vi "Insight_Write_Laser_Parameters_to_File.vi"(6 "Hold Data Vector":i32[](array[numeric]), 7 "Filename Preface (empty)":string, 8 "error in (no error)":errorcluster, 9 "Actual Laser Settings":T3={"Clock Rate (MHz)"=400.0, "Sample Pts"=0, "Total Sweep Pts"=0, "Total Pts Increment"=0, "Reversal Index"=0, "Sweep Efficiency (%)"=nan, "Duty Cycle (%)"=nan, "Repetition Rate (kHz)"=nan, "Sweep Rate (kHz)"=nan, "Min Wavelength (nm)"=nan, "Max Wavelength (nm)"=nan, "Power (mW)"=nan, "Power Profile"=enum."FLAT", "Edge Roll-off (dB)"=0.0, "Sample Clock Delay (nsec)"=0.0, "Sweep Start Delay (nsec)"=0.0, "Data Valid Delay (nsec)"=0.0, "Optical Freq. Step (GHz)"=0.1, "Sweep Start Trigger Edge"=enum."BOTH", "WL Sweep Direction?"=enum."Increase"}, 10 "Valid Vector":i32[](array[numeric]), 11 "Save Data Path":path=path "C:/Users/Demonstration/Documents/LabView_Applications/Projects/Insight_SPD_Acquire/laser_data") -> (0 "error out":errorcluster, 1 "Hold Data Vector Path":path=path "C:/Users/Demonstration/Documents/LabView_Applications/Projects/Insight_SPD_Acquire/laser_data", 2 "Laser Parameter Data Path":path=path "C:/Users/Demonstration/Documents/LabView_Applications/Projects/Insight_SPD_Acquire/laser_data", 3 "DVV Path":path=path "C:/Users/Demonstration/Documents/LabView_Applications/Projects/Insight_SPD_Acquire/laser_data")   [LabVIEW 2011]
doc: "Insight Photonic Solutions\n\nThis VI writes Actual Laser Settings cluster, Data Valid Vector and Hold Data Vector (aka Invalid Data Points) to Laser Parameter, DVV and Hold Data text files.\n\nUse the Filename Preface to add a specific filename descriptor like a date, time or random sequence.\n\nver 1.0 - original release\nver 1.1 - added inputs for the Hold Data Vector of hold points, writes this data to a file, and output the pathname to this file.\nver 3.5 - updated Actual Laser Settings to add Total Pts Incrementt, Reversal Index, and Sweep Rate. Also modified the formatting of the string written to the file to use the appropriate precision."
uses:
  Power_Profiles.ctl
  Start_Sweep_Trigger.ctl
  <vilib>/Utility/file.llb/Write To Spreadsheet File (I64).vi
  <vilib>/Utility/file.llb/Write To Spreadsheet File (string).vi
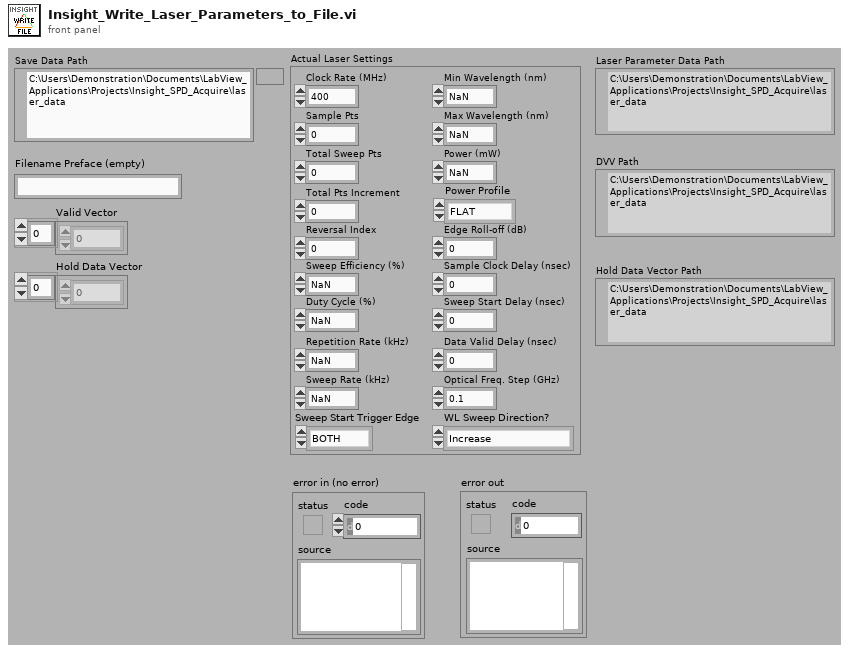
[diagram p1: front panel]
types:
  T1 = typedef "Power_Profiles.ctl" = enum16{"FLAT", "GAUSsian", "CUSTom"}
  T2 = typedef "Start_Sweep_Trigger.ctl" = enum16{"RISing", "FALLing", "BOTH"}
  T3 = cluster{"Clock Rate (MHz)":dbl, "Sample Pts":u32, "Total Sweep Pts":i32, "Total Pts Increment":i32, "Reversal Index":i32, "Sweep Efficiency (%)":dbl, "Duty Cycle (%)":dbl, "Repetition Rate (kHz)":dbl, "Sweep Rate (kHz)":dbl, "Min Wavelength (nm)":dbl, "Max Wavelength (nm)":dbl, "Power (mW)":dbl, "Power Profile":T1, "Edge Roll-off (dB)":dbl, "Sample Clock Delay (nsec)":dbl, "Sweep Start Delay (nsec)":dbl, "Data Valid Delay (nsec)":dbl, "Optical Freq. Step (GHz)":dbl, "Sweep Start Trigger Edge":T2, "WL Sweep Direction?":enum16{"Increase", "Decrease", "Bidirectional_Increase", "Bidirectional_Decrease"}}
  T4 = enum16{"Increase", "Decrease", "Bidirectional_Increase", "Bidirectional_Decrease"}
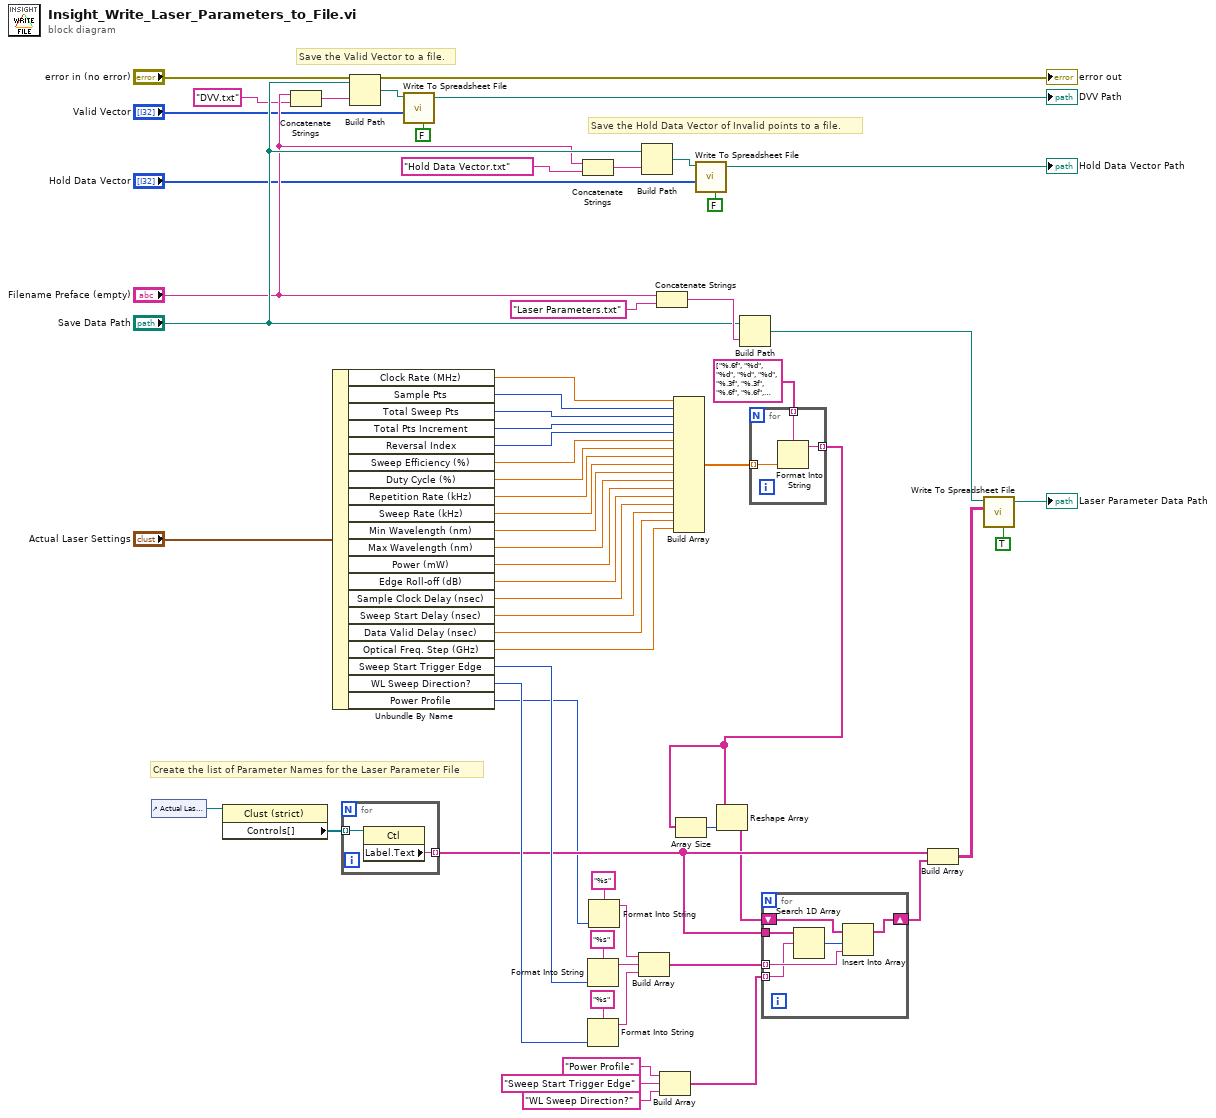
[diagram p0: block diagram]
diagram:
  # "Save the Hold Data Vector of Invalid points to a file."
  # "Save the Valid Vector to a file."
  # "Create the list of Parameter Names for the Laser Parameter File"
  n1 = control-ref of="Actual Laser Settings"() -> (w44:refnum<vi>)
  n2 = property class="Clust (strict)"(reference=w44) -> ("Controls[]"=w45:refnum<vi>[])  [unwired: 1 in, 2 out]
  n3 = Concatenate Strings("Filename Preface (empty)", "DVV.txt" ("time format string (%c)")) -> (w12:string)
  n4 = Unbundle By Name("Actual Laser Settings") -> ("Clock Rate (MHz)"=w62:dbl, "Sample Pts"=w61:u32, "Total Sweep Pts"=w60:i32, "Total Pts Increment"=w39:i32, "Reversal Index"=w38:i32, "Sweep Efficiency (%)"=w59:dbl, "Duty Cycle (%)"=w46:dbl, "Repetition Rate (kHz)"=w58:dbl, "Sweep Rate (kHz)"=w37:dbl, "Min Wavelength (nm)"=w57:dbl, "Max Wavelength (nm)"=w56:dbl, "Power (mW)"=w55:dbl, "Edge Roll-off (dB)"=w35:dbl, "Sample Clock Delay (nsec)"=w54:dbl, "Sweep Start Delay (nsec)"=w53:dbl, "Data Valid Delay (nsec)"=w52:dbl, "Optical Freq. Step (GHz)"=w51:dbl, "Sweep Start Trigger Edge"=w33:T2, "WL Sweep Direction?"=w31:T4, "Power Profile"=w2:T1)
  n5 = for {
    tunnel: w45 -> [w64] mode=indexing
    tunnel: [w63] -> w21 mode=indexing
    n6 = property class="Ctl"(reference=w64) -> ("Label.Text"=w63:string)  [unwired: 1 in, 2 out]
  }
  n7 = Build Path(base path="Save Data Path", name or relative path=w12) -> (appended path=w16:path)
  n8 = call-poly <vilib>:"Write To Spreadsheet File.vi"("transpose? (no:F)"=FALSE, "1D data"="Valid Vector", "file path (dialog if empty)"=w16) -> ("new file path (Not A Path if cancelled)"=→"DVV Path":path)  [unwired: 5 in]
  n9 = Concatenate Strings("Filename Preface (empty)", "Hold Data Vector.txt" ("time format string (%c)")) -> (w9:string)
  n10 = Format Into String(format string="%s", w33) -> (resulting string=w27:string)  [unwired: 2 in, 1 out]
  n11 = Format Into String(format string="%s", w31) -> (resulting string=w26:string)  [unwired: 2 in, 1 out]
  n12 = Format Into String(format string="%s", w2) -> (resulting string=w22:string)  [unwired: 2 in, 1 out]
  n13 = Build Array(w22, w27, w26) -> (w25:string[])
  n14 = Build Path(base path="Save Data Path", name or relative path=w9) -> (appended path=w7:path)
  n15 = Concatenate Strings("Filename Preface (empty)", "Laser Parameters.txt" ("time format string (%c)")) -> (w42:string)
  n16 = Build Array("Power Profile", "Sweep Start Trigger Edge", "WL Sweep Direction?") -> (w24:string[])
  n17 = Build Array(w62, w61, w60, w39, w38, w59, w46, w58, w37, w57, w56, w55, w35, w54, w53, w52, w51) -> (w49:dbl[])
  n18 = call-poly <vilib>:"Write To Spreadsheet File.vi"("transpose? (no:F)"=FALSE, "1D data"="Hold Data Vector", "file path (dialog if empty)"=w7) -> ("new file path (Not A Path if cancelled)"=→"Hold Data Vector Path":path)  [unwired: 5 in]
  n19 = Build Path(base path="Save Data Path", name or relative path=w42) -> (appended path=w48:path)
  n20 = for {
    tunnel: w49 -> [w67] mode=indexing
    tunnel: [w66] -> w1 mode=indexing
    tunnel: string[] ["%.6f", "%d", "%d", "%d", "%d", "%.3f", "%.3f", "%.6f", "%.6f", "%.4f", "%.4f", "%.3f", "%.3f", "%.3f", "%.3f", "%.3f", "%.6f"] -> [w65] mode=indexing
    n21 = Format Into String(format string=w65, w67) -> (resulting string=w66:string)  [unwired: 2 in, 1 out]
  }
  n22 = Array Size(array=w1) -> (size(s)=w20:i32)
  n23 = Reshape Array(w1, w20) -> (w19:string[])
  n24 = for {
    shift-right: [w72] -> w23
    shift-left: w19 -> [w71]
    tunnel: w25 -> [w70] mode=indexing
    tunnel: w21 -> [w69]
    tunnel: w24 -> [w68] mode=indexing
    n25 = Search 1D Array(1D array=w69, element=w68) -> (index of element=w73:i32)  [unwired: 1 in]
    n26 = Insert Into Array(array=w71, index=w73, new element=w70) -> (w72:string[])
  }
  n27 = Build Array(w21, w23) -> (w18:string[][])
  n28 = call-poly <vilib>:"Write To Spreadsheet File.vi"("transpose? (no:F)"=TRUE, "2D data"=w18, "file path (dialog if empty)"=w48) -> ("new file path (Not A Path if cancelled)"=→"Laser Parameter Data Path":path)  [unwired: 5 in]
  "error out" <- "error in (no error)"
